vi "Periodic Tasks.vi"(8 "error in":errorcluster) -> ()   [LabVIEW 2023]
doc: "This VI runs in parallel to other tasks. It can contain as many user-defined periodic loops as you need. These can carry out PID or other sorts of timed response."
uses:
  <vilib>/Rock Robotics/WPI/ThirdParty/Phoenix-LabVIEW/CANCoder/Get/CTRE_Phoenix_CANcoder_GetSensorData.vi
  <vilib>/Rock Robotics/Network Tables/NT Write Boolean.vi
  <vilib>/Rock Robotics/Network Tables/NT Write Number.vi
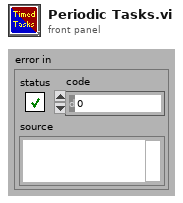
[diagram p1: front panel]
types:
  T1 = typedef "CTRE_Phoenix_CANcoder_DeviceRef.ctl" = cluster{"DeviceStatus":errorcluster, "Device Number":u8, "Handle":u64, "UsageFrame":u32, "Library Path":path}
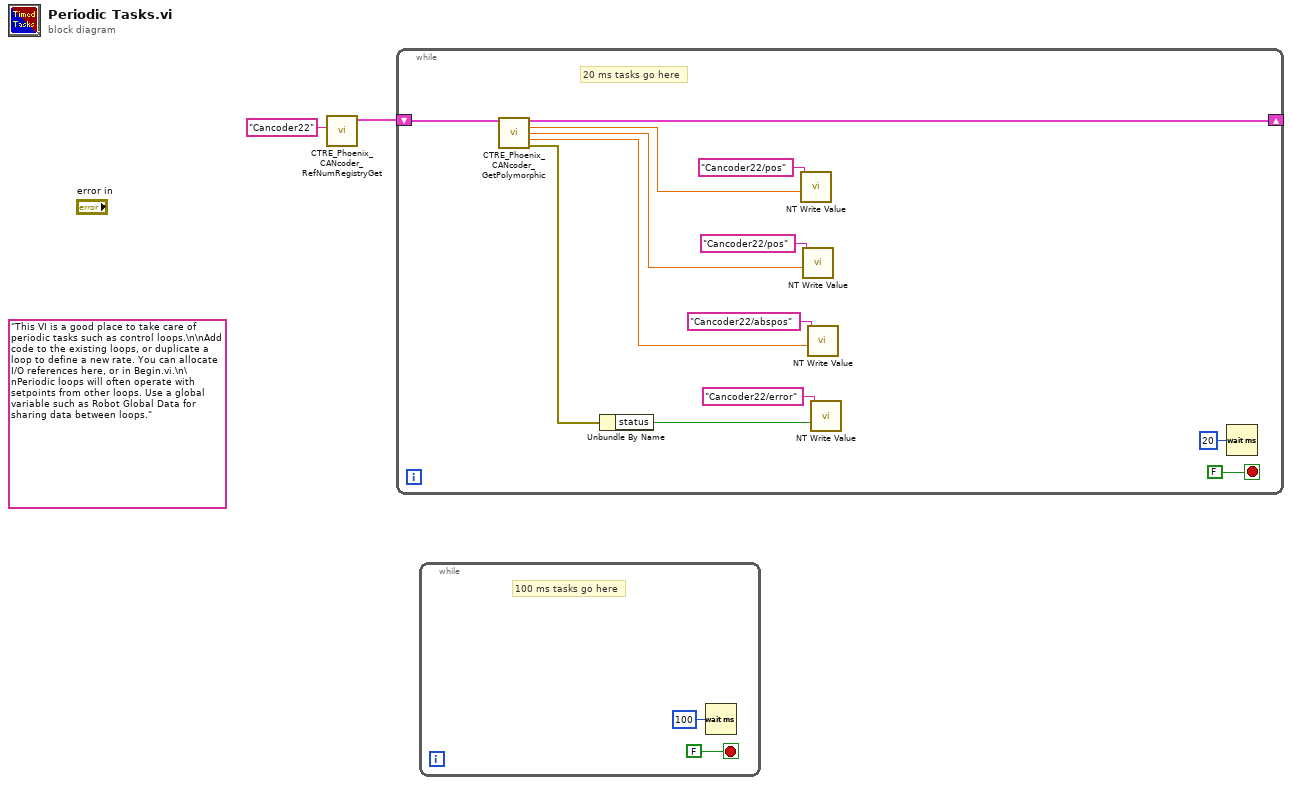
[diagram p0: block diagram]
diagram:
  (unwired) "This VI is a good place to take care of periodic tasks such as control loops.\n\nAdd code to the existing loops, or duplicate a loop to define a new rate. You can allocate I/O references here, or in Begin.vi.\n\nPeriodic loops will often operate with setpoints from other loops. Use a global variable such as Robot Global Data for sharing data between loops."
  n1 = call <vilib>:"CTRE_Phoenix_CANcoder_RefNumRegistryGet.vi"("refnum name"="Cancoder22") -> ("CTRE_CANcoder_DeviceRef"=w2:T1)  [unwired: 9 in, 1 out]
  n2 = while {
    shift-right: [w12] -> _
    shift-left: w2 -> [w13]
    stop <- FALSE stop-if-true
    # "20 ms tasks go here"
    n3 = call-poly <vilib>:"CTRE_Phoenix_CANcoder_GetPolymorphic.vi"("CTRE_CANcoder_DeviceRef"=w13) -> ("CTRE_CANcoder_DeviceRef"=w12:T1, "Position"=w7:dbl, "Velocity"=w6:dbl, "Absolute Position"=w5:dbl, "error out"=w4:errorcluster)  [unwired: 10 in]
    n4 = Unbundle By Name(w4) -> ("status"=w3:bool)
    n5 = call-poly <vilib>:"NT Write Value.vi"("value"=w7, "name"="Cancoder22/pos") -> ()  [unwired: 9 in, 1 out]
    n6 = call-poly <vilib>:"NT Write Value.vi"("value"=w6, "name"="Cancoder22/pos") -> ()  [unwired: 9 in, 1 out]
    n7 = call-poly <vilib>:"NT Write Value.vi"("value"=w5, "name"="Cancoder22/abspos") -> ()  [unwired: 9 in, 1 out]
    n8 = call-poly <vilib>:"NT Write Value.vi"("value"=w3, "name"="Cancoder22/error") -> ()  [unwired: 9 in, 1 out]
    n9 = Wait (ms)(milliseconds to wait=u32 20) -> ()  [unwired: 1 out]
  }
  n10 = while {
    stop <- FALSE stop-if-true
    # "100 ms tasks go here"
    n11 = Wait (ms)(milliseconds to wait=u32 100) -> ()  [unwired: 1 out]
  }
